vi "FTW-Crypto-FileHash.vi"(0 "Filepath":path, 5 "Algorithm":enum16{"SHA512", "SHA256", "SHA1", "MD5"}(ring), 7 "Hash Encoding":enum16{"No encoding", "Base64", "ASCII Hex"}(ring)=enum."ASCII Hex", 11 "error in":errorcluster) -> (4 "Filepath out":path, 6 "Hash out":string, 8 "Hash Length":i32, 10 "Filesize (bytes)":i64, 15 "error out":errorcluster)   [LabVIEW 2012]
panel:
  # "Inputs"
  # "Outputs"
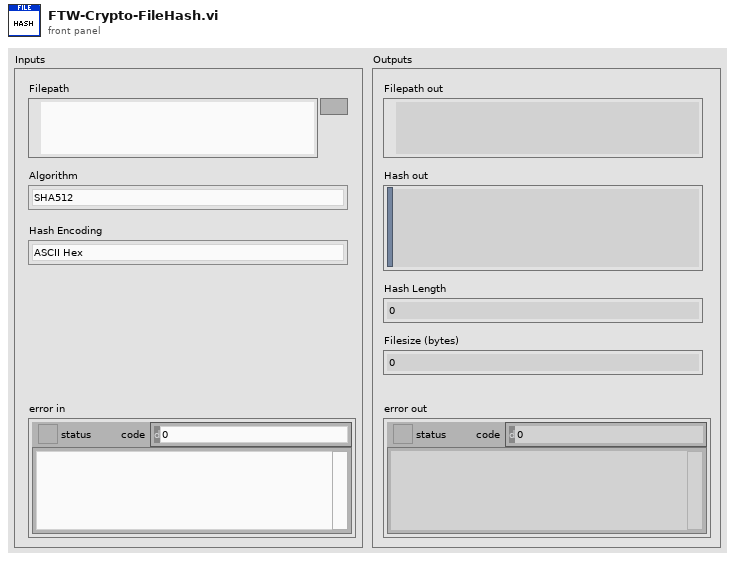
[diagram p1: front panel]
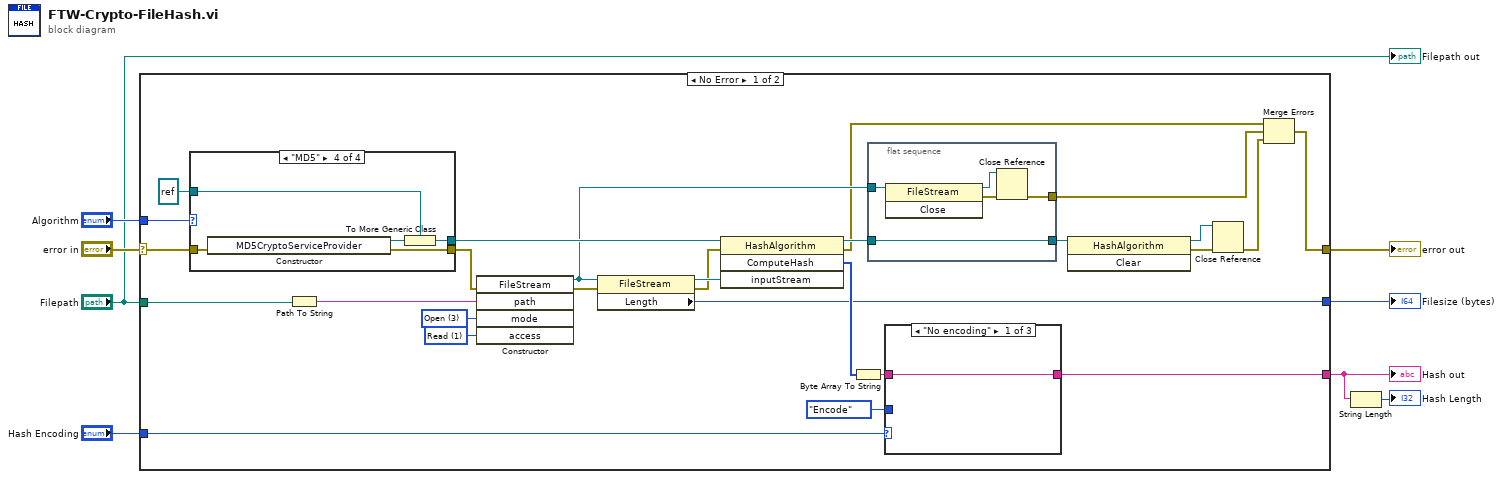
[diagram p0: block diagram]
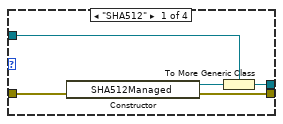
[diagram p2: hidden frame]
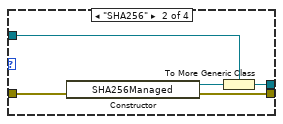
[diagram p3: hidden frame]
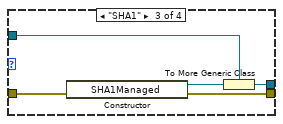
[diagram p4: hidden frame]
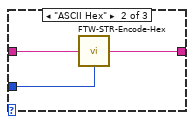
[diagram p5: hidden frame]
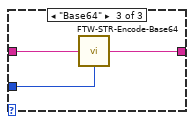
[diagram p6: hidden frame]
diagram:
  n1 = case shown="No Error" "error in" {
    selector: "error in" -> [w35 w68]
    tunnel: "Filepath" -> [w23 _]
    tunnel: [w30 _] -> w5
    tunnel: [w9 w68] -> w7
    tunnel: "Hash Encoding" -> [w32 _]
    tunnel: "Algorithm" -> [w28 _]
    tunnel: [w16 _] -> w2
    frame No Error {
      w24 = 3 items=["CreateNew"=1, "Create"=2, "Open"=3, "OpenOrCreate"=4, "Truncate"=5, "Append"=6] ("mode")
      w25 = 1 items=["Read"=1, "Write"=2, "ReadWrite"=3] ("access")
      n2 = case shown="\"MD5\"" w28 {
        tunnel: [w45 w50 w55 w60] -> w21
        tunnel: w35 -> [w44 w49 w54 w59]
        tunnel: [w42 w47 w52 w57] -> w26
        tunnel: refnum<k24> refnum (".NET Refnum") -> [w41 w46 w51 w56]
        frame "SHA512" {
          n3 = constructor class="SHA512Managed"(error in=w44) -> (reference out=w43:refnum<k24>, error out=w45:errorcluster)  [unwired: 2 in, 1 out]
          n4 = To More Generic Class(target class=w41, reference=w43) -> (generic class reference=w42:refnum<k24>)
        }
        frame "SHA256" {
          n5 = constructor class="SHA256Managed"(error in=w49) -> (reference out=w48:refnum<k24>, error out=w50:errorcluster)  [unwired: 2 in, 1 out]
          n6 = To More Generic Class(target class=w46, reference=w48) -> (generic class reference=w47:refnum<k24>)
        }
        frame "SHA1" {
          n7 = constructor class="SHA1Managed"(error in=w54) -> (reference out=w53:refnum<k24>, error out=w55:errorcluster)  [unwired: 2 in, 1 out]
          n8 = To More Generic Class(target class=w51, reference=w53) -> (generic class reference=w52:refnum<k24>)
        }
        frame "MD5" {
          n9 = constructor class="MD5CryptoServiceProvider"(error in=w59) -> (reference out=w58:refnum<k24>, error out=w60:errorcluster)  [unwired: 2 in, 1 out]
          n10 = To More Generic Class(target class=w56, reference=w58) -> (generic class reference=w57:refnum<k24>)
        }
      }
      n11 = Path To String(path=w23) -> (string=w22:string)
      n12 = constructor class="FileStream"(error in=w21, "path"=w22, "mode"=w24, "access"=w25) -> (reference out=w20:refnum<k24>, error out=w17:errorcluster)  [unwired: 2 in, 4 out]
      n13 = property class="FileStream"(reference=w20, error in=w17) -> (reference out=w19:refnum<k24>, error out=w18:errorcluster, "Length"=w16:i64)
      n14 = invoke class="HashAlgorithm" method="ComputeHash"(reference=w26, error in=w18, "inputStream"=w19) -> (reference out=w13:refnum<k24>, error out=w12:errorcluster, "ComputeHash"=w34:u8[])  [unwired: 1 in, 1 out]
      n15 = Byte Array To String(unsigned byte array=w34) -> (string=w31:string)
      n16 = flat-sequence {
        tunnel: w20 -> [w40]
        tunnel: [w37] -> w14
        tunnel: w13 -> [w37]
        tunnel: [w36] -> w11
        frame #0 {
          n17 = invoke class="FileStream" method="Close"(reference=w40) -> (reference out=w39:refnum<k24>, error out=w38:errorcluster)  [unwired: 2 in, 1 out]
          n18 = Close Reference(reference=w39, error in (no error)=w38) -> (error out=w36:errorcluster)
        }
      }
      n19 = case shown="\"No encoding\"" w32 {
        tunnel: w31 -> [w61 w64 w67]
        tunnel: [w61 w62 w66] -> w30
        tunnel: enum16{"Encode", "Decode"}."Encode" ("Direction") -> [_ w63 w65]
        frame "No encoding" {
        }
        frame "ASCII Hex" {
          n20 = call "FTW-STR-Encode-Hex.vi"("Input"=w64, "Direction"=w63) -> ("Output"=w62:string)
        }
        frame "Base64" {
          n21 = call "FTW-STR-Encode-Base64.vi"("Input"=w67, "Direction"=w65) -> ("Output"=w66:string)
        }
      }
      n22 = invoke class="HashAlgorithm" method="Clear"(reference=w14) -> (reference out=w33:refnum<k24>, error out=w15:errorcluster)  [unwired: 2 in, 1 out]
      n23 = Close Reference(reference=w33, error in (no error)=w15) -> (error out=w10:errorcluster)
      n24 = Merge Errors(w12, w11, w10) -> (w9:errorcluster)
    }
    frame Error {
    }
  }
  "Hash out" <- w5
  "error out" <- w7
  "Filesize (bytes)" <- w2
  n25 = String Length(string=w5) -> (length=→"Hash Length":i32)
  "Filepath out" <- "Filepath"
